vi "Backup By Varying MultiplesOfBytes.vi"(7 "Backup on Size Multiples (Bytes)":i32[](array[numeric])=[67, 300, 10000], 8 "error in":errorcluster, 9 "Label (VI Title)":string="Memory on various BackUp - Check", 10 "Test Sequence Condition Checked":string[](array[string])=["Frequent Backup for every Data being inserted", "Normal Backup for every 5 times of Data being inserted", "Leisure Backup, for once in a Blue moon for Max Data inserted"], 11 "TableLogger Config":T1={"TableLogger"=enum."SQLite Logger", "DB File Path"=path "DB.db", "DB Backup Config"={"Directory"=path "DB/Backup", "UTC Time Format"=FALSE, "On Launch"=FALSE, "Interval (Hours)"=100.0, "Size Multiples (Bytes)"=24}}) -> (0 "error out":errorcluster)   [LabVIEW 2014]
uses:
  TableLogger_Actor/TableLoggerConfig.ctl
  TableLogger_Actor/TableLoggerTypes.ctl
  TableLogger_Actor/TableLoggerBackupConfig.ctl
  TableLogger_Actor/TableLogger_Actor.lvlib
panel:
  # "1, Frequent - each line of Small Data inserted takes 67 Bytes in memory\n2, Normal - 4 or 5 times of inserting 67 Bytes in memory\n3, Leisure - 10K bytes once backup taken"
  # "Connector Pane"
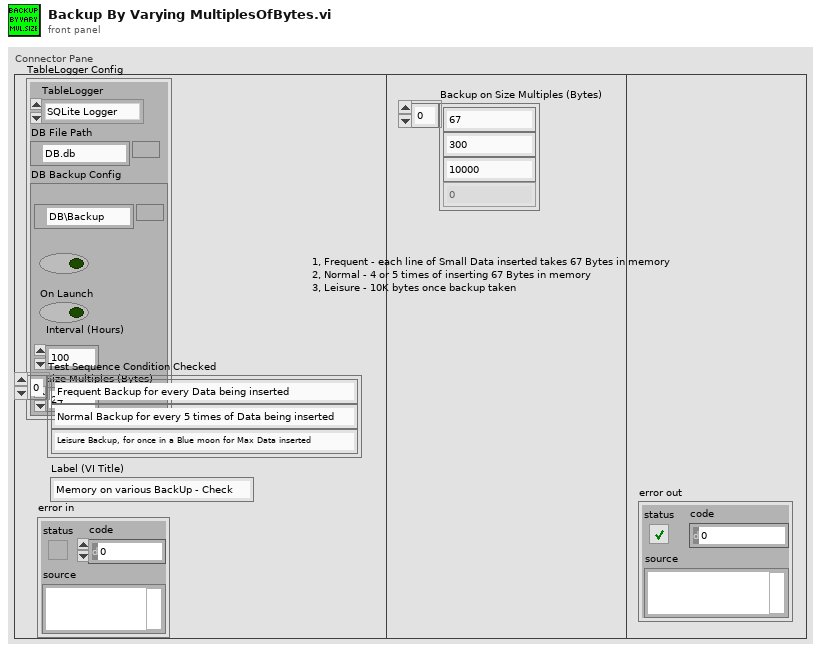
[diagram p1: front panel]
types:
  T1 = typedef "TableLogger_Actor.lvlib/TableLoggerConfig.ctl" = cluster{"TableLogger":T2, "DB File Path":path, "DB Backup Config":T3}
  T2 = typedef "TableLogger_Actor.lvlib/TableLoggerTypes.ctl" = enum16{"CSV Logger", "SQLite Logger"}
  T3 = typedef "TableLogger_Actor.lvlib/TableLoggerBackupConfig.ctl" = cluster{"Directory":path, "UTC Time Format":bool, "On Launch":bool, "Interval (Hours)":dbl, "Size Multiples (Bytes)":i32}
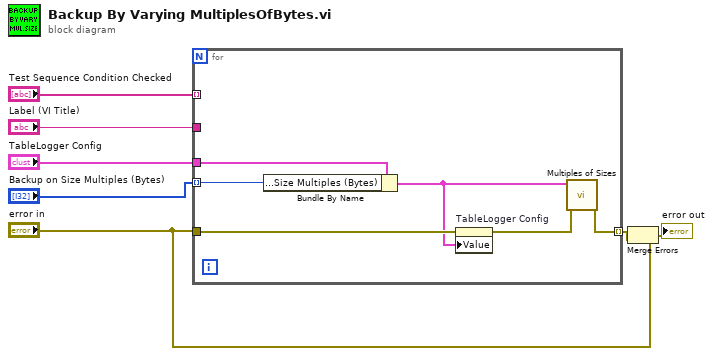
[diagram p0: block diagram]
diagram:
  n1 = for {
    tunnel: "TableLogger Config" -> [w13]
    tunnel: "Backup on Size Multiples (Bytes)" -> [w12] mode=indexing
    tunnel: "Test Sequence Condition Checked" -> [_] mode=indexing
    tunnel: "error in" -> [w10]
    tunnel: [w11] -> w4 mode=indexing
    tunnel: "Label (VI Title)" -> [_]
    n2 = Bundle By Name(cluster=w13, "DB Backup Config.Size Multiples (Bytes)"=w12) -> (w8:T1)
    n3 = property on="TableLogger Config" class="Clust (strict)"(error in=w10, "Value"=w8) -> (error out=w9:errorcluster)  [unwired: 1 in, 1 out]
    n4 = call "Multiples of Sizes.vi"("error in"=w9, "TableLogger Config"=w8) -> ("error out"=w11:errorcluster)  [unwired: 9 in]
  }
  n5 = Merge Errors("error in", w4) -> (→"error out":errorcluster)
